vi "DIselector.vi"(8 "I/O element":T1(ring)) -> (3 "value":bool)   [LabVIEW 2023]
uses:
  <vilib>/eio/EIONode/EIONode.xnode
  <vilib>/rvi/eio/common/nirviEmuTemplateMethod_errors.vi
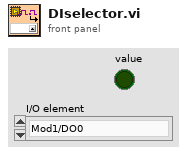
[diagram p1: front panel]
types:
  T1 = enum16{"Mod1/DO0", "Mod1/DO1", "Mod1/DO2", "Mod1/DO3", "Mod1/DO4", "Mod1/DO5", "Mod1/DO6", "Mod1/DO7", "Mod4/DIO0", "Mod4/DIO1", "Mod4/DIO2", "Mod4/DIO3", "Mod4/DIO4", "Mod4/DIO5", "Mod4/DIO6", "Mod4/DIO7", "Mod6/DIO0", "Mod6/DIO1", "Mod6/DIO2", "Mod6/DIO3", "Mod6/DIO4", "Mod6/DIO5", "Mod6/DIO6", "Mod6/DIO7"}
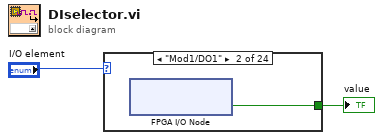
[diagram p0: block diagram]
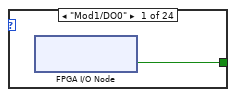
[diagram p2: hidden frame]
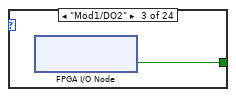
[diagram p3: hidden frame]
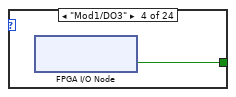
[diagram p4: hidden frame]
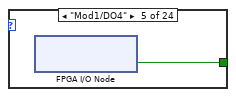
[diagram p5: hidden frame]
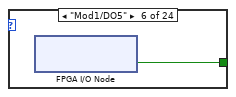
[diagram p6: hidden frame]
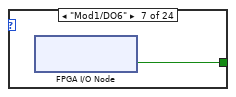
[diagram p7: hidden frame]
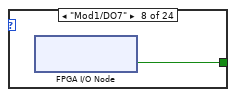
[diagram p8: hidden frame]
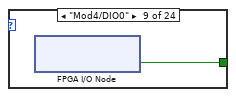
[diagram p9: hidden frame]
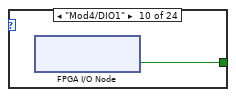
[diagram p10: hidden frame]
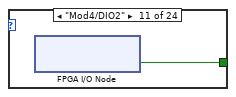
[diagram p11: hidden frame]
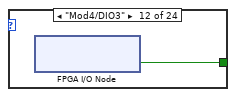
[diagram p12: hidden frame]
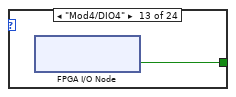
[diagram p13: hidden frame]
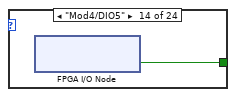
[diagram p14: hidden frame]
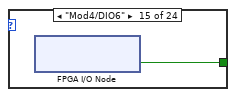
[diagram p15: hidden frame]
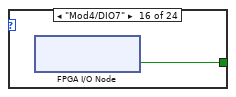
[diagram p16: hidden frame]
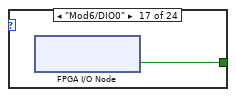
[diagram p17: hidden frame]
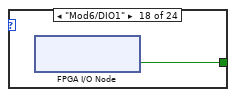
[diagram p18: hidden frame]
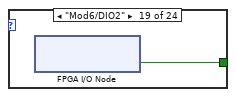
[diagram p19: hidden frame]
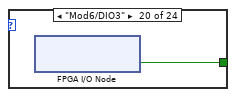
[diagram p20: hidden frame]
diagram:
  n1 = case shown="\"Mod1/DO1\"" "I/O element" {
    tunnel: [w3 w4 w5 w6 w7 w8 w9 w10 w11 w12 w13 w14 w15 w16 w17 w18 w19 w20 w21 w22 w23 w24 w25 w26] -> w1
    frame "Mod1/DO0" {
      n2 = xnode "FPGA I/O Node"() -> ("Mod1/DO0"=w3:bool)  [unwired: 1 in, 1 out]
    }
    frame "Mod1/DO1" {
      n3 = xnode "FPGA I/O Node"() -> ("Mod1/DO1"=w4:bool)  [unwired: 1 in, 1 out]
    }
    frame "Mod1/DO2" {
      n4 = xnode "FPGA I/O Node"() -> ("Mod1/DO2"=w5:bool)  [unwired: 1 in, 1 out]
    }
    frame "Mod1/DO3" {
      n5 = xnode "FPGA I/O Node"() -> ("Mod1/DO3"=w6:bool)  [unwired: 1 in, 1 out]
    }
    frame "Mod1/DO4" {
      n6 = xnode "FPGA I/O Node"() -> ("Mod1/DO4"=w7:bool)  [unwired: 1 in, 1 out]
    }
    frame "Mod1/DO5" {
      n7 = xnode "FPGA I/O Node"() -> ("Mod1/DO5"=w8:bool)  [unwired: 1 in, 1 out]
    }
    frame "Mod1/DO6" {
      n8 = xnode "FPGA I/O Node"() -> ("Mod1/DO6"=w9:bool)  [unwired: 1 in, 1 out]
    }
    frame "Mod1/DO7" {
      n9 = xnode "FPGA I/O Node"() -> ("Mod1/DO7"=w10:bool)  [unwired: 1 in, 1 out]
    }
    frame "Mod4/DIO0" {
      n10 = xnode "FPGA I/O Node"() -> ("Mod4/DIO0"=w11:bool)  [unwired: 1 in, 1 out]
    }
    frame "Mod4/DIO1" {
      n11 = xnode "FPGA I/O Node"() -> ("Mod4/DIO1"=w12:bool)  [unwired: 1 in, 1 out]
    }
    frame "Mod4/DIO2" {
      n12 = xnode "FPGA I/O Node"() -> ("Mod4/DIO2"=w13:bool)  [unwired: 1 in, 1 out]
    }
    frame "Mod4/DIO3" {
      n13 = xnode "FPGA I/O Node"() -> ("Mod4/DIO3"=w14:bool)  [unwired: 1 in, 1 out]
    }
    frame "Mod4/DIO4" {
      n14 = xnode "FPGA I/O Node"() -> ("Mod4/DIO4"=w15:bool)  [unwired: 1 in, 1 out]
    }
    frame "Mod4/DIO5" {
      n15 = xnode "FPGA I/O Node"() -> ("Mod4/DIO5"=w16:bool)  [unwired: 1 in, 1 out]
    }
    frame "Mod4/DIO6" {
      n16 = xnode "FPGA I/O Node"() -> ("Mod4/DIO6"=w17:bool)  [unwired: 1 in, 1 out]
    }
    frame "Mod4/DIO7" {
      n17 = xnode "FPGA I/O Node"() -> ("Mod4/DIO7"=w18:bool)  [unwired: 1 in, 1 out]
    }
    frame "Mod6/DIO0" {
      n18 = xnode "FPGA I/O Node"() -> ("Mod6/DIO0"=w19:bool)  [unwired: 1 in, 1 out]
    }
    frame "Mod6/DIO1" {
      n19 = xnode "FPGA I/O Node"() -> ("Mod6/DIO1"=w20:bool)  [unwired: 1 in, 1 out]
    }
    frame "Mod6/DIO2" {
      n20 = xnode "FPGA I/O Node"() -> ("Mod6/DIO2"=w21:bool)  [unwired: 1 in, 1 out]
    }
    frame "Mod6/DIO3" {
      n21 = xnode "FPGA I/O Node"() -> ("Mod6/DIO3"=w22:bool)  [unwired: 1 in, 1 out]
    }
    frame "Mod6/DIO4" {
      n22 = xnode "FPGA I/O Node"() -> ("Mod6/DIO4"=w23:bool)  [unwired: 1 in, 1 out]
    }
    frame "Mod6/DIO5" {
      n23 = xnode "FPGA I/O Node"() -> ("Mod6/DIO5"=w24:bool)  [unwired: 1 in, 1 out]
    }
    frame "Mod6/DIO6" {
      n24 = xnode "FPGA I/O Node"() -> ("Mod6/DIO6"=w25:bool)  [unwired: 1 in, 1 out]
    }
    frame "Mod6/DIO7" {
      n25 = xnode "FPGA I/O Node"() -> ("Mod6/DIO7"=w26:bool)  [unwired: 1 in, 1 out]
    }
  }
  "value" <- w1
